vi "Path gen.vi"(8 "error in (no error)":errorcluster, 10 "Path":path, 11 "Generador in":refnum<class "Generador.lvclass">) -> (0 "error out":errorcluster, 3 "Generador out":refnum<class "Generador.lvclass">)   [LabVIEW 2020, in "Generador señal.lvlib" / "Generador.lvclass"]
uses:
  Generador.lvclass
  Generador.lvclass/Generador.ctl
  Text File/Text File Messages/Write Path Msg/Write Path Msg.lvclass/Write Path Msg.ctl
  <vilib>/ActorFramework/Message Enqueuer/Message Enqueuer.lvclass/Message Enqueuer.ctl
  <vilib>/ActorFramework/Message Enqueuer/Enqueue.vi
  Text File/Text File Messages/Write Path Msg/Write Path Msg.lvclass
  C:/Program Files (x86)/National Instruments/LabVIEW 2020/vi.lib/ActorFramework/Message/Message.lvclass
  <vilib>/ActorFramework/Message Priority Queue/Priority Enqueue.vi
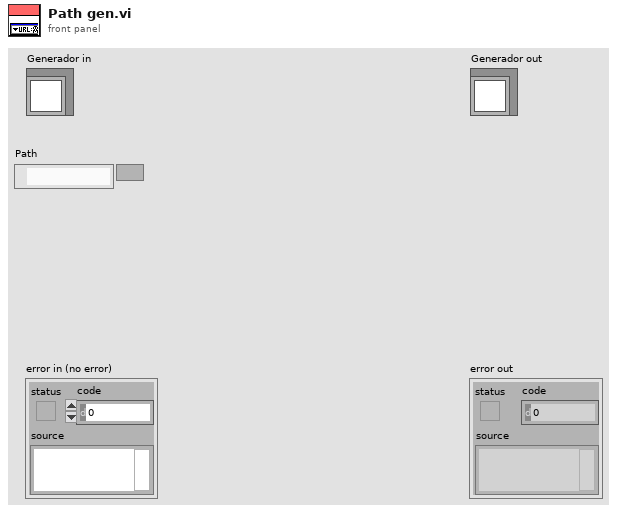
[diagram p1: front panel]
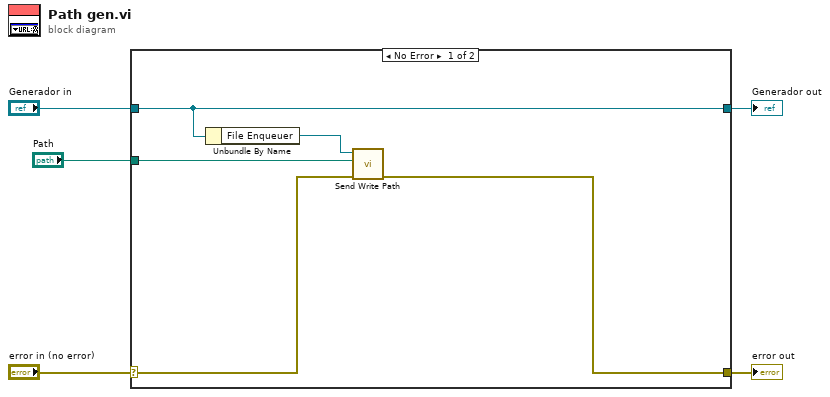
[diagram p0: block diagram]
diagram:
  n1 = case shown="No Error" "error in (no error)" {
    selector: "error in (no error)" -> [w7 w12]
    tunnel: [w6 w12] -> w4
    tunnel: [w9 w11] -> w2
    tunnel: "Generador in" -> [w9 w11]
    tunnel: "Path" -> [w8 _]
    frame No Error {
      n2 = Unbundle By Name(w9) -> ("File Enqueuer"=w10:refnum<class "Message Enqueuer.lvclass">)
      n3 = call "Send Write Path.vi"("error in (no error)"=w7, "Path"=w8, "Message Enqueuer"=w10) -> ("error out"=w6:errorcluster)  [unwired: 7 in, 1 out]
    }
    frame Error {
    }
  }
  "error out" <- w4
  "Generador out" <- w2
